vi "Read Voltage.vi"   [LabVIEW 2020, in "Keithley 2600 Series.lvlib"]
doc: "Performs a current sweep with voltage measured at every point."
uses:
  <instrlib>/Keithley 2600 Series/Keithley 2600 Series.lvlib
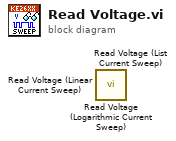
[diagram p0: block diagram]
diagram:
  n1 = call <instrlib>:"Read Voltage (Logarithmic Current Sweep).vi"() -> ()  [unwired: 9 in, 3 out]
  n2 = call <instrlib>:"Read Voltage (List Current Sweep).vi"() -> ()  [unwired: 9 in, 3 out]
  n3 = call <instrlib>:"Read Voltage (Linear Current Sweep).vi"() -> ()  [unwired: 9 in, 3 out]
